vi "DatReadParams.vi"(6 "error in (no error)":errorcluster, 7 "default Values":dbl[](array[numeric])=[1.0, 2.0], 8 "Names":string[](array[string])=["par1", "par2"], 9 "tracename":string="F:\\2017 10 06\\current vi's\\Data\\data_025.tdms: 2") -> (0 "error out":errorcluster, 1 "Values out":dbl[](array[numeric])=[1.0, 2.0], 3 "tracename out":string)   [LabVIEW 2018]
uses:
  <vilib>/Utility/file.llb/Read From Spreadsheet File (string).vi
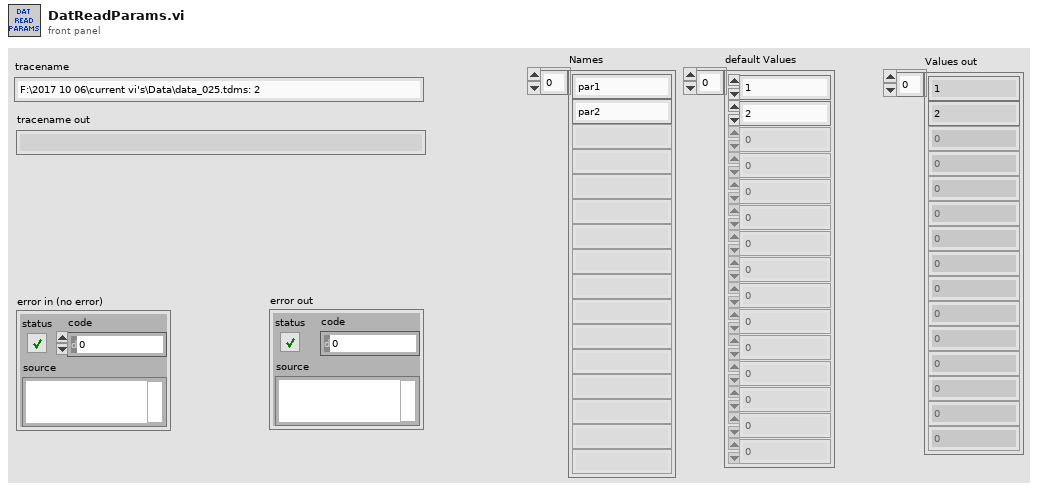
[diagram p1: front panel]
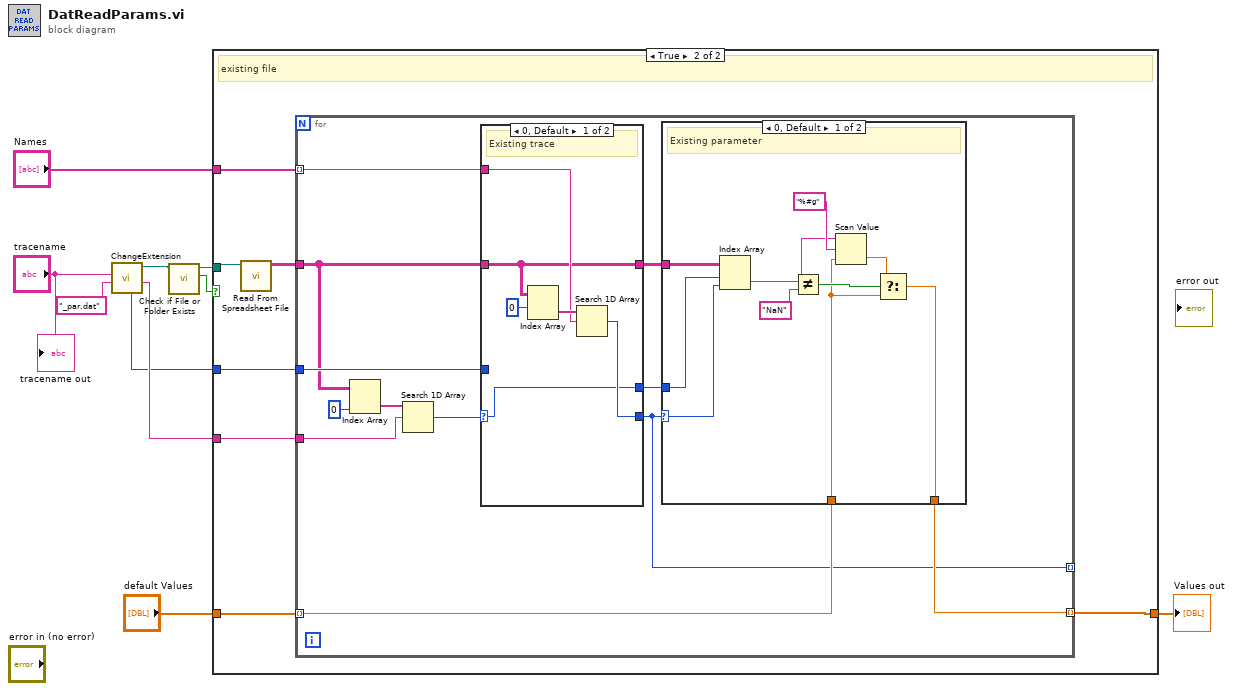
[diagram p0: block diagram]
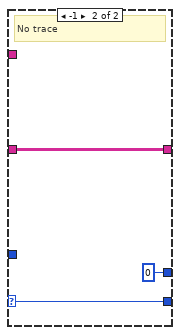
[diagram p4: hidden frame]
diagram:
  n1 = call "ChangeExtension.vi"("extension"="_par.dat", "file in"="tracename") -> (1:"Tracenr"=w5:string, "Path out"=w7:path, 4:"Tracenr"=w3:i32)  [unwired: 3 in, 2 out]
  n2 = call <vilib>:"Check if File or Folder Exists.vi"("path"=w7) -> ("file or folder exists?"=w4:bool, "dup path"=w6:path)  [unwired: 8 in, 1 out]
  n3 = case shown="True" w4 {
    tunnel: "Names" -> [_ w18]
    tunnel: w6 -> [_ w15]
    tunnel: w5 -> [_ w17]
    tunnel: w3 -> [_ w16]
    tunnel: [w11 w12] -> w2
    tunnel: "default Values" -> [w11 w14]
    frame False {
      # "No file"
    }
    frame True {
      # "existing file"
      n4 = call-poly <vilib>:"Read From Spreadsheet File.vi"("file path (dialog if empty)"=w15) -> ("all rows"=w13:string[][])  [unwired: 6 in, 4 out]
      n5 = for {
        tunnel: w18 -> [w25] mode=indexing
        tunnel: w17 -> [w26]
        tunnel: w16 -> [w28]
        tunnel: w14 -> [w21] mode=indexing
        tunnel: w13 -> [w24]
        tunnel: [w20] -> w12 mode=indexing
        tunnel: [w19] -> _ mode=indexing
        n6 = Index Array(array=w24, index (col)=0 ("disabled index (col)")) -> (element=w27:string[])  [unwired: 1 in]
        n7 = Search 1D Array(1D array=w27, element=w26) -> (index of element=w29:i32)  [unwired: 1 in]
        n8 = case shown="0, Default" w29 {
          selector: w29 -> [w43 w50]
          tunnel: [w44 w50] -> w19
          tunnel: w28 -> [_ _]
          tunnel: w25 -> [w45 _]
          tunnel: w24 -> [w42 w49]
          tunnel: [w43 0 ("index of element")] -> w22
          tunnel: [w42 w49] -> w23
          frame 0, Default {
            # "Existing trace"
            n9 = Index Array(array=w42, index (row)=0) -> (element=w47:string[])  [unwired: 1 in]
            n10 = Search 1D Array(1D array=w47, element=w45) -> (index of element=w44:i32)  [unwired: 1 in]
          }
          frame -1 {
            # "No trace"
          }
        }
        n11 = case shown="0, Default" w19 {
          selector: w19 -> [w38 _]
          tunnel: w23 -> [w40 _]
          tunnel: w22 -> [w39 _]
          tunnel: w21 -> [w32 w41]
          tunnel: [w31 w41] -> w20
          frame 0, Default {
            # "Existing parameter"
            n12 = Index Array(array=w40, index (row)=w39, index (col)=w38) -> (element=w36:string)
            n13 = Not Equal?(x=w36, y="NaN") -> (x != y?=w34:bool)
            n14 = Scan Value(string=w36, format string="%#g", default (0 dbl)=w32) -> (value=w33:dbl)  [unwired: 1 out]
            n15 = Select(t=w33, s=w34, f=w32) -> (s? t:f=w31:dbl)
          }
          frame -1 {
            # "No parameter"
          }
        }
      }
    }
  }
  "Values out" <- w2
  "tracename out" <- "tracename"
